vi "Fill Slider Values.vi"(10 "LBCB Number":T3, 11 "DofType":T2) -> (2 "Silder Values":T1(array[cluster]))   [LabVIEW 2009]
uses:
  Data Access Objects/Metadata/LBCB Number.ctl
  Data Access Objects/Limits/DofTypes.ctl
  Data Access Objects/Metadata/Persistant DAO Actions.ctl
panel:
  in  "Values":string[](array[string])=["Global Lower", "Global Higher", "Local Lower", "Local Higher", "Global Actual", "Local Actual"]
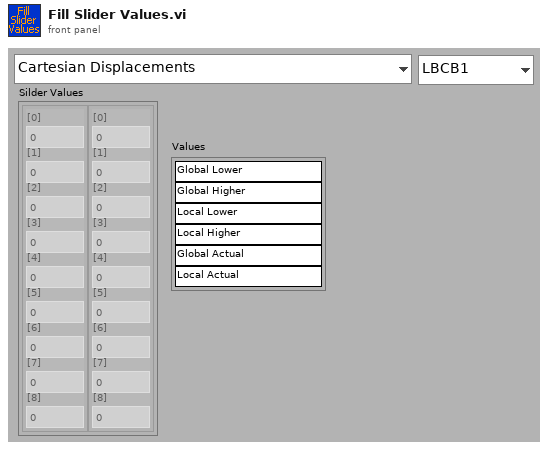
[diagram p1: front panel]
types:
  T1 = cluster{"[0]":dbl, "[1]":dbl, "[2]":dbl, "[3]":dbl, "[4]":dbl, "[5]":dbl, "[6]":dbl, "[7]":dbl, "[8]":dbl}[]
  T2 = typedef "DofTypes.ctl" = enum16{"Cartesian Displacements", "Cartesian Forces & Moments", "Actuator Displacements", "Actuator Forces", "Cartesian Increments", "Actuator Increments"}
  T3 = typedef "LBCB Number.ctl" = enum16{"LBCB1", "LBCB2"}
  T4 = typedef "Persistant DAO Actions.ctl" = enum16{"Init", "Get", "Set", "Load", "Save"}
  T5 = typedef "Dataset Source.ctl" = enum16{"LBCB 1", "LBCB 2", "Combined", "External Sensors"}
  T6 = typedef "Actuator Matrix.ctl" = cluster{"Lower":T7, "Upper":T7}
  T7 = typedef "Actuator Point.ctl" = cluster{"X1":dbl, "X2":dbl, "Y1":dbl, "Z1":dbl, "Z2":dbl, "Z3":dbl}
  T8 = typedef "Cartesian Point.ctl" = cluster{"Dx":dbl, "Dy":dbl, "Dz":dbl, "Rx":dbl, "Ry":dbl, "Rz":dbl}
  T9 = typedef "Cartesian Matrix.ctl" = cluster{"Lower":T8, "Upper":T8}
  T10 = typedef "Act & Cart Commands.ctl" = cluster{"Act Cmd":dbl[], "Cart Cmd":dbl[]}
  T11 = typedef "Limit Matrix.ctl" = dbl[][]
  T12 = cluster{"[0]":dbl, "[1]":dbl, "[2]":dbl, "[3]":dbl, "[4]":dbl, "[5]":dbl, "[6]":dbl, "[7]":dbl, "[8]":dbl}[][]
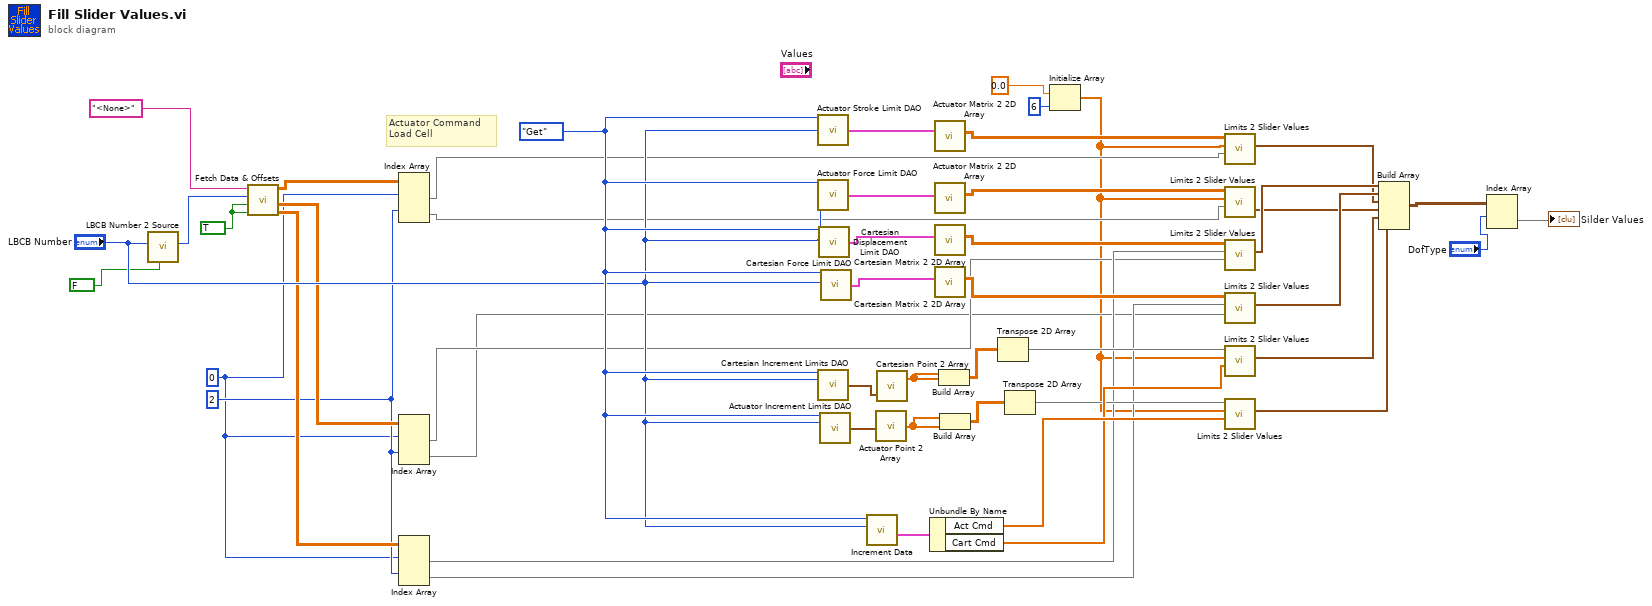
[diagram p0: block diagram]
diagram:
  w2 = TRUE ("Include Command")
  w7 = 2 ("index")
  w6 = 0 ("index (row)")
  w25 = Persistant_DAO_Actions."Get" ("Actuator Stroke Limit Actions")
  # "Actuator Command\nLoad Cell"
  n1 = call "LBCB Number 2 Source.vi"("Combined"=FALSE, "LBCB Number"="LBCB Number") -> ("Dataset Source"=w12:T5)  [unwired: 9 in]
  n2 = call "Fetch Data & Offsets.vi"("Include Command"=w2, "Include Reading"=w2, "Source"=w12, "Force Tag"="<None>") -> ("Cartesian Offsets"=w8:dbl[][], "Cartesian Data"=w9:dbl[][], "Actuator Data"=w10:dbl[][])  [unwired: 1 out]
  n3 = Index Array(array=w10, index (row) #1=w6, index (row) #2=w7) -> (element #1=w16:dbl[], element #2=w15:dbl[])  [unwired: 2 in]
  n4 = Index Array(array=w9, index (row) #1=w6, index (row) #2=w7) -> (element #1=w5:dbl[], element #2=w4:dbl[])  [unwired: 2 in]
  n5 = Index Array(array=w8, index (row) #1=w6, index (row) #2=w7) -> (element #1=w14:dbl[], element #2=w13:dbl[])  [unwired: 2 in]
  n6 = call "Actuator Stroke Limit DAO.vi"("Actuator Stroke Limit Actions"=w25, "ID"="LBCB Number") -> ("Actuator Stroke Limits Out"=w48:T6)  [unwired: 11 in, 2 out]
  n7 = call "Actuator Force Limit DAO.vi"("Actuator Force Limit Actions"=w25, "ID"="LBCB Number") -> ("Actuator Force Limits Out"=w47:T6)  [unwired: 11 in, 2 out]
  n8 = call "Cartesian Increment Limits DAO.vi"("Actions"=w25, "LBCB Number"="LBCB Number") -> ("Inc Limits Out"=w33:T8)  [unwired: 11 in, 2 out]
  n9 = call "Cartesian Displacement Limit DAO.vi"("Cartesian Displacement Limit Actions"=w25, "ID"="LBCB Number") -> ("Cartesian Displacement Out"=w46:T9)  [unwired: 11 in, 2 out]
  n10 = call "Actuator Increment Limits DAO.vi"("Actions"=w25, "LBCB Number"="LBCB Number") -> ("Inc Limits Out"=w32:T7)  [unwired: 11 in, 2 out]
  n11 = call "Cartesian Force Limit DAO.vi"("Cartesian Force Limit Actions"=w25, "ID"="LBCB Number") -> ("Cartesian Force Limit Out"=w45:T9)  [unwired: 11 in, 2 out]
  n12 = call "Increment Data.vi"("LBCB Number"="LBCB Number", "DAO Actions"=w25) -> ("Increments Out"=w24:T10)  [unwired: 8 in, 1 out]
  n13 = call "Actuator Point 2 Array.vi"("Actuator Point"=w32) -> ("Array"=w30:dbl[])
  n14 = call "Cartesian Point 2 Array.vi"("Cart Disp"=w33) -> ("Array"=w31:dbl[])  [unwired: 2 in]
  n15 = Unbundle By Name(w24) -> ("Act Cmd"=w23:dbl[], "Cart Cmd"=w22:dbl[])
  n16 = call "Actuator Matrix 2 2D Array.vi"("Matrix In"=w48) -> ("Matrix Out"=w44:T11)  [unwired: 10 in]
  n17 = call "Actuator Matrix 2 2D Array.vi"("Matrix In"=w47) -> ("Matrix Out"=w43:T11)  [unwired: 10 in]
  n18 = call "Cartesian Matrix 2 2D Array.vi"("Matrix In"=w46) -> ("Matrix Out"=w42:T11)  [unwired: 10 in]
  n19 = call "Cartesian Matrix 2 2D Array.vi"("Matrix In"=w45) -> ("Matrix Out"=w41:T11)  [unwired: 10 in]
  n20 = Build Array(w31, w31) -> (w29:dbl[][])
  n21 = Build Array(w30, w30) -> (w28:dbl[][])
  n22 = Transpose 2D Array(2D array=w29) -> (transposed array=w19:dbl[][])
  n23 = Transpose 2D Array(2D array=w28) -> (transposed array=w18:dbl[][])
  n24 = Initialize Array(0.0 ("element"), 6 ("dimension size")) -> (w1:dbl[])
  n25 = call "Limits 2 Slider Values.vi"("Actual"=w16, "Offsets"=w1, "Limits"=w44) -> ("Values"=w38:T1)  [unwired: 8 in]
  n26 = call "Limits 2 Slider Values.vi"("Actual"=w15, "Offsets"=w1, "Limits"=w43) -> ("Values"=w37:T1)  [unwired: 8 in]
  n27 = call "Limits 2 Slider Values.vi"("Actual"=w5, "Offsets"=w14, "Limits"=w42) -> ("Values"=w40:T1)  [unwired: 8 in]
  n28 = call "Limits 2 Slider Values.vi"("Actual"=w4, "Offsets"=w13, "Limits"=w41) -> ("Values"=w39:T1)  [unwired: 8 in]
  n29 = call "Limits 2 Slider Values.vi"("Actual"=w22, "Offsets"=w1, "Limits"=w19) -> ("Values"=w21:T1)  [unwired: 8 in]
  n30 = call "Limits 2 Slider Values.vi"("Actual"=w23, "Offsets"=w1, "Limits"=w18) -> ("Values"=w20:T1)  [unwired: 8 in]
  n31 = Build Array(w40, w39, w38, w37, w21, w20) -> (w36:T12)
  n32 = Index Array(array=w36, index (row)="DofType") -> (element=→"Silder Values":T1)  [unwired: 1 in]
